vi "日期时间字符串转换分钟数加一.vi"(10 "枚举":enum16{"分钟数加一", "秒数加一", "小时数加一"}(ring), 11 "data[0]":string) -> (3 "日期/时间字符串":string)   [LabVIEW 2016, in "数据传输系统-02.lvlib"]
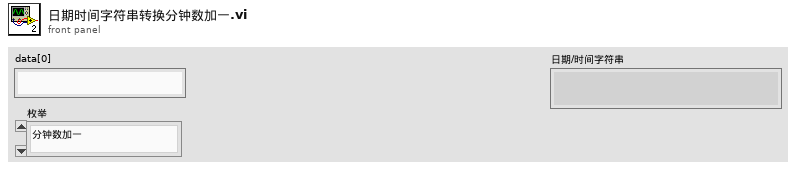
[diagram p1: front panel]
types:
  T1 = typedef "LVDateTimeRec.ctl" = cluster{"秒数的小数部分":dbl, "秒":i32, "分":i32, "时":i32, "日":i32, "月":i32, "年":i32, "天数（周）":i32, "天数（年）":i32, "DST":i32}
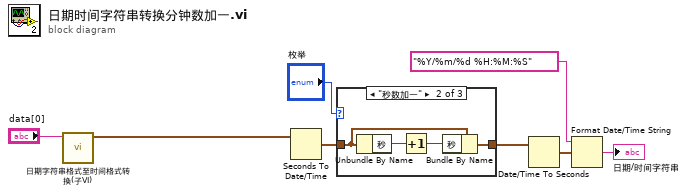
[diagram p0: block diagram]
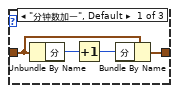
[diagram p2: hidden frame]
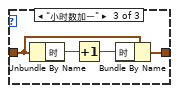
[diagram p3: hidden frame]
diagram:
  n1 = call "日期字符串格式至时间格式转换(子VI).vi"("data[0]"="data[0]") -> ("time stamp"=w4:timestamp)  [unwired: 10 in]
  n2 = Seconds To Date/Time(time stamp (now)=w4) -> (date time rec=w5:T1)  [unwired: 1 in]
  n3 = case shown="\"秒数加一\"" "枚举" {
    tunnel: [w12 w13 w17] -> w7
    tunnel: w5 -> [w10 w14 w18]
    frame "分钟数加一", Default {
      n4 = Unbundle By Name(w10) -> ("分"=w9:i32)
      n5 = Increment(x=w9) -> (x+1=w11:i32)
      n6 = Bundle By Name(cluster=w10, "分"=w11) -> (w12:T1)
    }
    frame "秒数加一" {
      n7 = Unbundle By Name(w14) -> ("秒"=w15:i32)
      n8 = Increment(x=w15) -> (x+1=w16:i32)
      n9 = Bundle By Name(cluster=w14, "秒"=w16) -> (w13:T1)
    }
    frame "小时数加一" {
      n10 = Unbundle By Name(w18) -> ("时"=w19:i32)
      n11 = Increment(x=w19) -> (x+1=w20:i32)
      n12 = Bundle By Name(cluster=w18, "时"=w20) -> (w17:T1)
    }
  }
  n13 = Date/Time To Seconds(2:w7) -> (0:w6:timestamp)  [unwired: 1 in]
  n14 = Format Date/Time String(time format string (%c)="%Y/%m/%d %H:%M:%S" ("时间格式字符串(%c)"), seconds (now)=w6) -> (date/time string=→"日期/时间字符串":string)  [unwired: 1 in]
